vi "XY Graph Transpose Plot Event.vi"(8 "Error In":errorcluster, 11 "Mouse Click Event Data":T1) -> (0 "Error Out":errorcluster, 1 "Message":string, 3 "Plot Name":string, 5 "Graph Caption":string)   [LabVIEW 2021, in "XY Graph Add-Ons.lvlib"]
uses:
  XY Graph Add-Ons.lvlib
  XY Graph Mouse Click Event Data.ctl
  XY Graph Refnum.ctl
  <vilib>/Utility/miscctls.llb/LVPoint32TypeDef.ctl
  Get Plot at Mouse Click (XY Graph)/Get Plot at Mouse Click [AAC].vi
  XY Graph Add Single Plot with Name.vi
  Graphs.lvlib
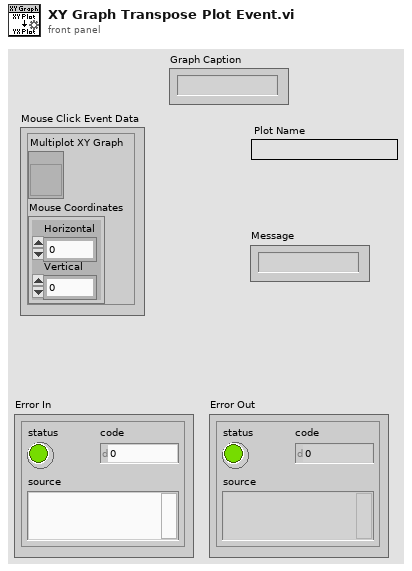
[diagram p1: front panel]
types:
  T1 = typedef "XY Graph Add-Ons.lvlib/XY Graph Mouse Click Event Data.ctl" = cluster{"Multiplot XY Graph":T2, "Mouse Coordinates":T3}
  T2 = typedef "XY Graph Add-Ons.lvlib/XY Graph Refnum.ctl" = refnum<vi>
  T3 = typedef "LVPoint32TypeDef.ctl" = cluster{"Horizontal":i32, "Vertical":i32}
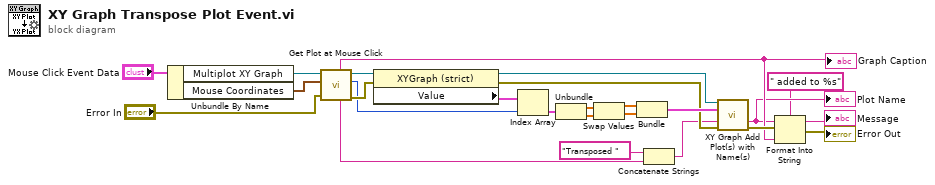
[diagram p0: block diagram]
diagram:
  n1 = Unbundle By Name("Mouse Click Event Data") -> ("Multiplot XY Graph"=w24:T2, "Mouse Coordinates"=w23:T3)
  n2 = call-poly "Get Plot at Mouse Click.vi"("error in (no error)"="Error In", "Mouse Click Coordinates"=w23, "XYGraph Ref"=w24) -> ("error out"=w20:errorcluster, "Plot at Coordinates"=w18:i32, "XYGraph Ref"=w21:T2, "Plot Name"=w3:string, "Graph Name"=w14:string)  [unwired: 2 in, 2 out]
  "Graph Caption" <- w14
  n3 = property class="XYGraph (strict)"(reference=w21, error in=w20) -> (reference out=w16:T2, error out=w5:errorcluster, "Value"=w19:cluster{"X Array":dbl[], "Y Array":dbl[]}[])
  n4 = Index Array(array=w19, index=w18) -> (element=w17:cluster{"X Array":dbl[], "Y Array":dbl[]})
  n5 = Unbundle(w17) -> ("X Array"=w10:dbl[], "Y Array"=w9:dbl[])
  n6 = Swap Values(12:w10, 14:w9) -> (1:w8:dbl[], 3:w7:dbl[])  [unwired: 1 in]
  n7 = Bundle(w8, w7) -> (w6:cluster{dbl[], dbl[]})  [unwired: 1 in]
  n8 = Concatenate Strings("Transposed " ("initial string"), w3) -> (w2:string)
  n9 = call-poly "XY Graph Add Plot(s) with Name(s).vi"("XYGraph Ref in"=w16, "Plot"=w6, "Plot Name (\"Plot\")"=w2, "error in (no error)"=w5) -> ("Plot Name"=w12:string, "error out"=w15:errorcluster)  [unwired: 8 in, 2 out]
  "Plot Name" <- w12
  n10 = Format Into String(format string=" added to %s", initial string=w12, error in=w15, w14) -> (resulting string=→"Message":string, error out=→"Error Out":errorcluster)
